vi "Update Control from Metadata.vi"(6 "default_value":variant, 8 "error in":errorcluster, 9 "control name":string, 10 "parameter data":T1[](array[typedef]), 11 "vi refnum":refnum<vi>) -> (0 "error out":errorcluster)   [LabVIEW 2021, in "NI Measurement V2 Client Generator Runtime.lvlib"]
uses:
  NI Measurement V2 Client Generator Runtime.lvlib
  <vilib>/gRPC/Generated APIs/ni/measurementlink/measurement/v2/Measurement Service Client V2/RPC Messages/ni_measurementlink_measurement_v2_ConfigurationParameter.ctl
  <vilib>/gRPC/Generated APIs/ni/measurementlink/measurement/v2/Measurement Service Client V2/RPC Messages/google_protobuf_Field_Kind.ctl
  <vilib>/gRPC/Generated APIs/ni/measurementlink/measurement/v2/Measurement Service Client V2/RPC Messages/ni_measurementlink_measurement_v2_ConfigurationParameter_AnnotationsEntry.ctl
  <vilib>/Utility/miscctls.llb/LVPositionTypeDef.ctl
  Client Generator Error Strings Global.vi
  <vilib>/gRPC/Generated APIs/ni/measurementlink/measurement/v2/Measurement Service Client V2/Measurement Service Client V2.lvlib
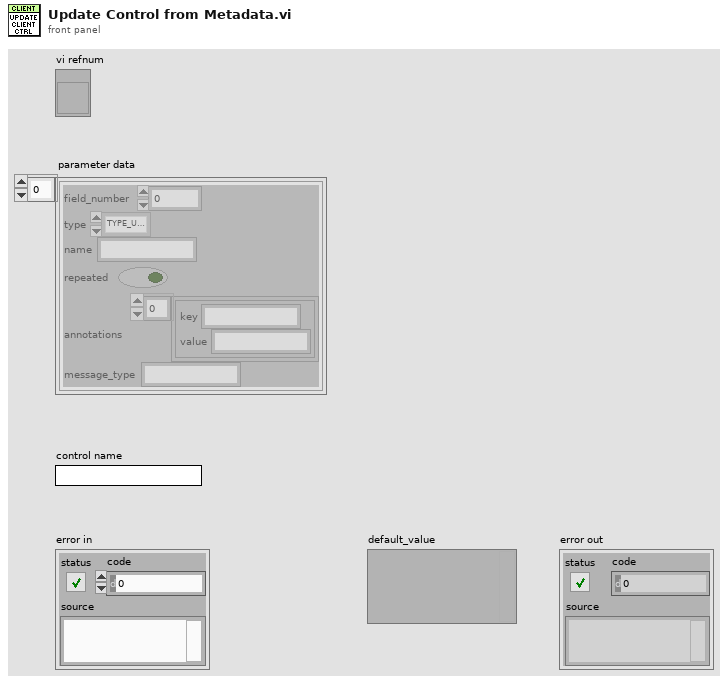
[diagram p1: front panel]
types:
  T1 = typedef "Measurement Service Client V2.lvlib/ni_measurementlink_measurement_v2_ConfigurationParameter.ctl" = cluster{"field_number":i32, "type":T2, "name":string, "repeated":bool, "annotations":T3[], "message_type":string}
  T2 = typedef "Measurement Service Client V2.lvlib/google_protobuf_Field_Kind.ctl" = enum32{"TYPE_UNKNOWN", "TYPE_DOUBLE", "TYPE_FLOAT", "TYPE_INT64", "TYPE_UINT64", "TYPE_INT32", "TYPE_FIXED64", "TYPE_FIXED32", "TYPE_BOOL", "TYPE_STRING", "TYPE_GROUP", "TYPE_MESSAGE", "TYPE_BYTES", "TYPE_UINT32", "TYPE_ENUM", "TYPE_SFIXED32", "TYPE_SFIXED64", "TYPE_SINT32", "TYPE_SINT64"}
  T3 = typedef "Measurement Service Client V2.lvlib/ni_measurementlink_measurement_v2_ConfigurationParameter_AnnotationsEntry.ctl" = cluster{"key":string, "value":string}
  T4 = typedef "LVPositionTypeDef.ctl" = cluster{"Left":i32, "Top":i32}
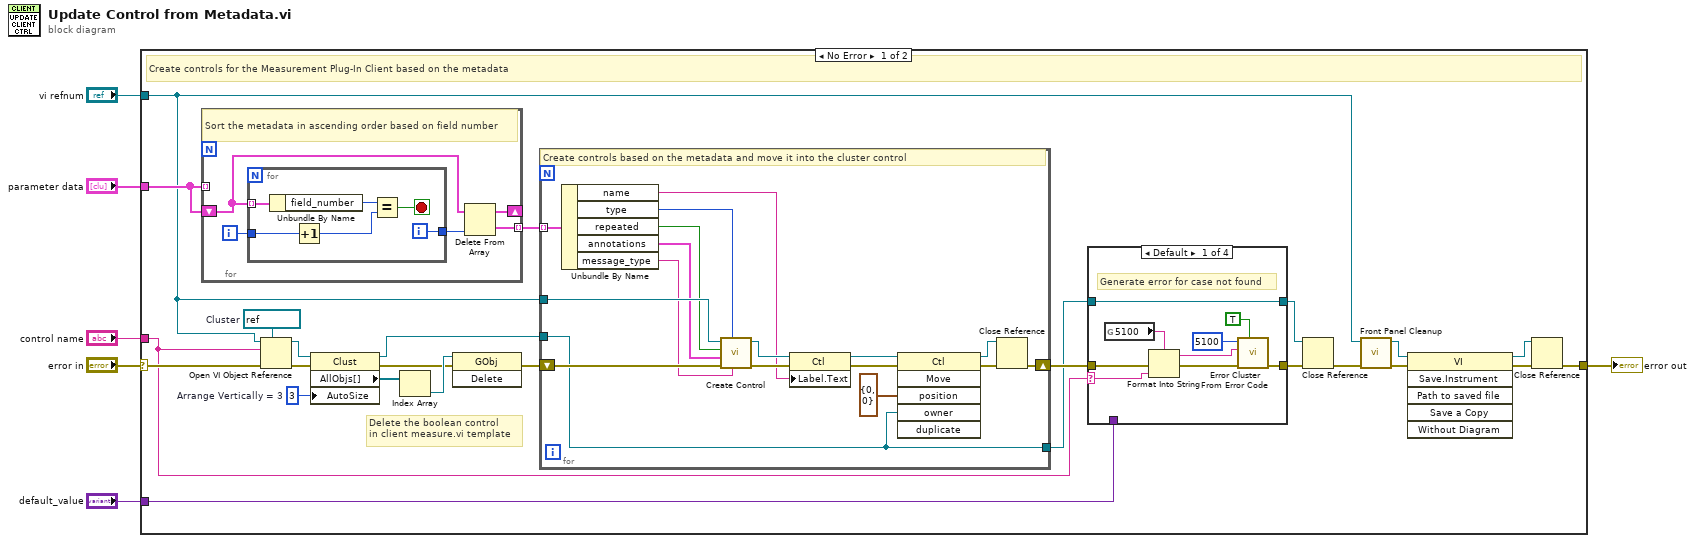
[diagram p0: block diagram]
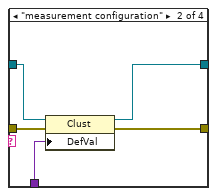
[diagram p2: hidden frame]
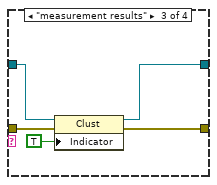
[diagram p3: hidden frame]
diagram:
  n1 = case shown="No Error" "error in" {
    selector: "error in" -> [w25 w81]
    tunnel: "control name" -> [w18 _]
    tunnel: "parameter data" -> [w16 _]
    tunnel: "vi refnum" -> [w8 _]
    tunnel: [w12 w81] -> w3
    tunnel: "default_value" -> [w11 _]
    frame No Error {
      w24 = u32 3  # Arrange Vertically = 3
      w31 = refnum<vi> refnum  # Cluster
      # "Delete the boolean control\nin client measure.vi template"
      # "Create controls for the Measurement Plug-In Client based on the metadata"
      n2 = for {
        shift-right: [w50] -> _
        shift-left: w16 -> [w51]
        tunnel: [w49] -> w17 mode=indexing
        tunnel: w16 -> [_] mode=indexing
        i -> [w53]
        # "Sort the metadata in ascending order based on field number"
        n3 = for {
          tunnel: w51 -> [w56] mode=indexing
          tunnel: w53 -> [w59]
          tunnel: [w55] -> w52
          i -> [w55]
          stop <- w54 stop-if-true
          n4 = Unbundle By Name(w56) -> ("field_number"=w58:i32)
          n5 = Increment(x=w59) -> (x+1=w57:i32)
          n6 = Equal?(x=w58, y=w57) -> (x = y?=w54:bool)
        }
        n7 = Delete From Array(array=w51, index=w52) -> (deleted portion=w49:T1, array with subset deleted=w50:T1[])  [unwired: 1 in]
      }
      n8 = Open VI Object Reference(7:w31, 8:w25, 10:w18, 11:w8) -> (0:w29:errorcluster, 3:w30:refnum<vi>)
      n9 = property class="Clust"(reference=w30, error in=w29, "AutoSize"=w24) -> (reference out=w21:refnum<vi>, error out=w26:errorcluster, "AllObjs[]"=w28:refnum<vi>[])
      n10 = Index Array(array=w28) -> (element=w27:refnum<vi>)  [unwired: 1 in]
      n11 = invoke class="GObj" method="Delete"(reference=w27, error in=w26) -> (error out=w23:errorcluster)  [unwired: 1 in, 2 out]
      n12 = for {
        shift-right: [w36] -> w22
        shift-left: w23 -> [w48]
        tunnel: w8 -> [w46]
        tunnel: w21 -> [w34]
        tunnel: [w34] -> w19
        tunnel: w17 -> [w32] mode=indexing
        # "Create controls based on the metadata and move it into the cluster control"
        n13 = Unbundle By Name(w32) -> ("name"=w40:string, "type"=w44:T2, "repeated"=w45:bool, "annotations"=w43:T3[], "message_type"=w42:string)
        n14 = call "Create Control.vi"("message_type"=w42, "type"=w44, "error in"=w48, "annotations"=w43, "is repeated?"=w45, "vi refnum"=w46) -> ("error out"=w47:errorcluster, "control ref"=w41:refnum<vi>)  [unwired: 4 in]
        n15 = property class="Ctl"(reference=w41, error in=w47, "Label.Text"=w40) -> (reference out=w39:refnum<vi>, error out=w38:errorcluster)
        n16 = invoke class="Ctl" method="Move"(reference=w39, error in=w38, "position"=T4 {"Left"=0, "Top"=0}, "owner"=w34) -> (reference out=w35:refnum<vi>, error out=w37:errorcluster)  [unwired: 2 in, 4 out]
        n17 = Close Reference(reference=w35, error in (no error)=w37) -> (error out=w36:errorcluster)
      }
      n18 = case shown="Default" w18 {
        selector: w18 -> [w63 _ _ _]
        tunnel: w22 -> [w68 w73 w78 w79]
        tunnel: [w66 w72 w77 w79] -> w20
        tunnel: w19 -> [w67 w71 w76 w80]
        tunnel: [w67 w70 w75 w80] -> w10
        tunnel: w11 -> [_ w69 _ _]
        frame Default {
          # "Generate error for case not found"
          n19 = global read "Client Generator Error Strings Global.vi" "5100"() -> (w60:string)
          n20 = Format Into String(format string=w60, error in=w68, w63) -> (resulting string=w61:string, error out=w64:errorcluster)  [unwired: 1 in]
          n21 = call <vilib>:"Error Cluster From Error Code.vi"("show call chain? (False)"=TRUE, "error in (no error)"=w64, "error message (\"\")"=w61, "error code (0)"=5100) -> ("error out"=w66:errorcluster)  [unwired: 5 in]
        }
        frame "measurement configuration" {
          n22 = property class="Clust"(reference=w71, error in=w73, "DefVal"=w69) -> (reference out=w70:refnum<vi>, error out=w72:errorcluster)
        }
        frame "measurement results" {
          n23 = property class="Clust"(reference=w76, error in=w78, "Indicator"=TRUE) -> (reference out=w75:refnum<vi>, error out=w77:errorcluster)
        }
        frame "configuration" {
        }
      }
      n24 = Close Reference(reference=w10, error in (no error)=w20) -> (error out=w13:errorcluster)
      n25 = call "Front Panel Cleanup.vi"("error in"=w13, "vi refnum"=w8) -> ("error out"=w9:errorcluster, "vi refnum out"=w7:refnum<vi>)  [unwired: 8 in]
      n26 = invoke class="VI" method="Save.Instrument"(reference=w7, error in=w9) -> (reference out=w15:refnum<vi>, error out=w14:errorcluster)  [unwired: 4 in, 4 out]
      n27 = Close Reference(reference=w15, error in (no error)=w14) -> (error out=w12:errorcluster)
    }
    frame Error {
      # "Pass"
    }
  }
  "error out" <- w3
